vi "Initialize Work.vi"(8 "error in (no error)":errorcluster, 9 "Cycle period":dbl, 10 "Reply to":refnum<class "Result Reply Msg.lvclass">, 11 "Measure Controller in":refnum<class "Process Controller.lvclass">) -> (0 "error out":errorcluster, 3 "Measure Controller out":refnum<class "Process Controller.lvclass">)   [LabVIEW 2016, in "Process Controller.lvclass"]
uses:
  Process Controller.lvclass
  Template Module Messages/Result Reply Msg/Result Reply Msg.lvclass
  Process Controller Messages/Init Response Msg/Init Response Msg.lvclass
  C:/github/Measure_core/Template Module Messages/Result Reply Msg/Result Reply Msg.lvclass
  Results/Acquired Result/Acquired Result.lvclass
  Worker Messages/Initialize Work Msg/Initialize Work Msg.lvclass/Initialize Work Msg.ctl
  <vilib>/ActorFramework/Message Enqueuer/Message Enqueuer.lvclass/Message Enqueuer.ctl
  Process Controller.lvclass/Process Controller.ctl
  <vilib>/ActorFramework/Message Enqueuer/Enqueue.vi
  Worker Messages/Initialize Work Msg/Initialize Work Msg.lvclass
  C:/Program Files/National Instruments/LabVIEW 2016/vi.lib/ActorFramework/Message/Message.lvclass
  <vilib>/ActorFramework/Message Priority Queue/Priority Enqueue.vi
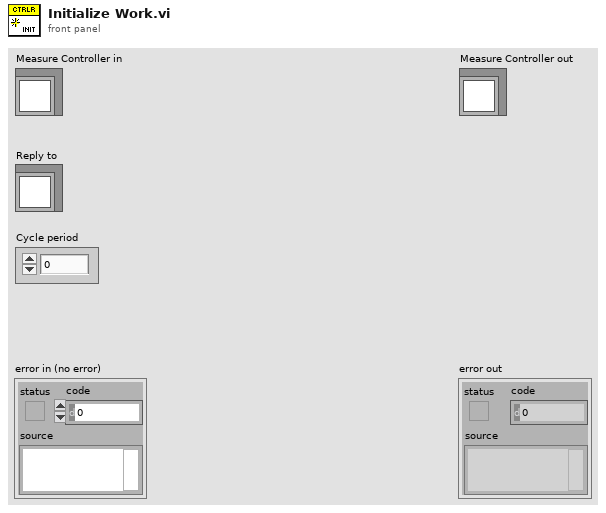
[diagram p1: front panel]
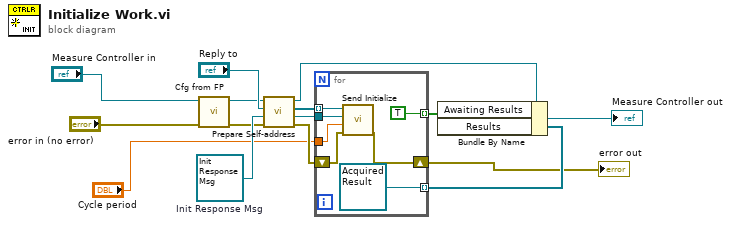
[diagram p0: block diagram]
diagram:
  w6 = refnum<class "Init Response Msg.lvclass"> refnum  # Init Response Msg
  n1 = call-dynamic "Cfg from FP.vi"("error in (no error)"="error in (no error)", "Measure Object in"="Measure Controller in") -> ("error out"=w4:errorcluster, "Measure Object out"=w2:refnum<class "Process Controller.lvclass">)  [unwired: 8 in]
  n2 = call-dynamic "Prepare Self-address.vi"("error in (no error)"=w4, "Reply to me"=w6, "Reply to"="Reply to", "Measure Controller in"=w2) -> ("error out"=w8:errorcluster, "Reply to me"=w10:refnum<class "Result Reply Msg.lvclass">, "Active measurements enqueuers"=w9:refnum<class "Message Enqueuer.lvclass">[], "Measure Controller out"=w7:refnum<class "Process Controller.lvclass">)  [unwired: 4 in]
  n3 = for {
    tunnel: w9 -> [w18] mode=indexing
    shift-right: [w22] -> w12
    shift-left: w8 -> [w17]
    tunnel: [TRUE] -> w15 mode=indexing
    tunnel: [refnum<class "Acquired Result.lvclass"> refnum ("Placeholder Result")] -> w14 mode=indexing
    tunnel: w10 -> [w19]
    tunnel: "Cycle period" -> [w16]
    n4 = call "Send Initialize.vi"("error in (no error)"=w17, "Cycle period"=w16, "Reply to"=w19, "Message Enqueuer"=w18) -> ("error out"=w22:errorcluster)  [unwired: 6 in, 1 out]
  }
  "error out" <- w12
  n5 = Bundle By Name(cluster=w7, "Awaiting Results"=w15, "Results"=w14) -> (→"Measure Controller out":refnum<class "Process Controller.lvclass">)
